vi "NS Width.vi"(10 "m-nm WB":dbl, 11 "Width of Base":dbl) -> (3 "Numeric":dbl)   [LabVIEW 2020]
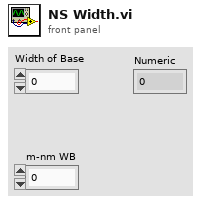
[diagram p1: front panel]
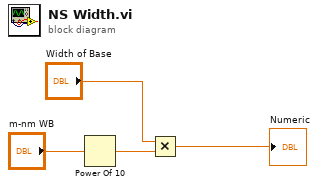
[diagram p0: block diagram]
diagram:
  n1 = Power Of 10(x="m-nm WB") -> (10^x=w2:dbl)
  n2 = Multiply(x="Width of Base", y=w2) -> (x*y=→"Numeric":dbl)
